vi "Obtain Broadcast Events.vi"(8 "error in":errorcluster, 10 "Create New? (F)":bool) -> (0 "error out":errorcluster, 2 "Main HMI Broadcast Events":T1)   [LabVIEW 2021, in "Main HMI.lvlib"]
doc: "This VI Obtains/Creates the Broadcast events that will be used for other modules to register to receive messages from the module that owns this VI.\n\n<b>NOTE</b>: The contents of this VI are automatically generated and modified by the <b>Tools > DQMH Consortium > DQMH</b> utilities. Consider using those utilities instead of making your own modifications to this VI.\n_____\nBased on DQMH Dev Tools: Project Template 7.1.2.1547."
uses:
  Main HMI.lvlib
  Broadcast Events--cluster.ctl
  Did Init Argument--cluster.ctl
  Status Updated Argument--cluster.ctl
  Error Reported Argument--cluster.ctl
  Stop Argument--cluster.ctl
  Get Module Execution Status Argument--cluster.ctl
panel:
  # "NOTE: The contents of this VI are automatically generated and modified by the Tools > DQMH Consortium > DQMH utilities. Consider using those utilities instead of making your own modifications to this VI."
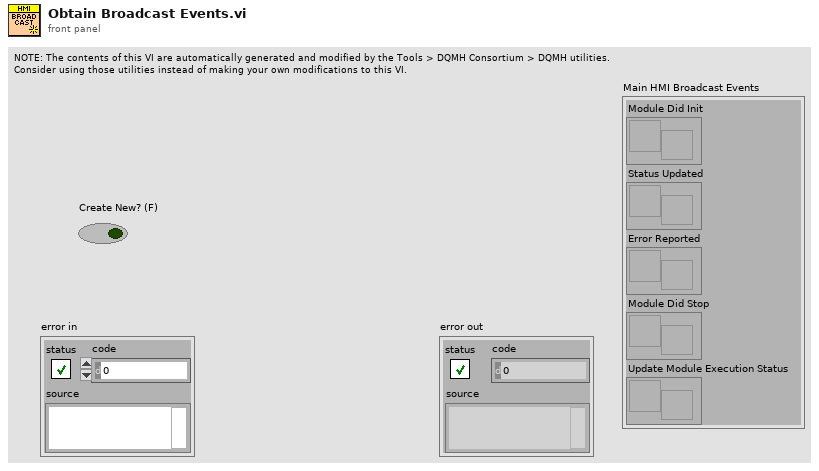
[diagram p1: front panel]
types:
  T1 = typedef "Main HMI.lvlib/Broadcast Events--cluster.ctl" = cluster{"Module Did Init":refnum<user-event>, "Status Updated":refnum<user-event>, "Error Reported":refnum<user-event>, "Module Did Stop":refnum<user-event>, "Update Module Execution Status":refnum<user-event>}
  T2 = typedef "Main HMI.lvlib/Get Module Execution Status Argument--cluster.ctl" = cluster{"Running?":bool}
  T3 = typedef "Main HMI.lvlib/Stop Argument--cluster.ctl" = cluster{"Origin":string, "Exit via Stop Module Req?":bool, "Wait for Module to stop?":bool}
  T4 = typedef "Main HMI.lvlib/Error Reported Argument--cluster.ctl" = cluster{"Error":errorcluster, "Additional Information":string, "Module Name":string}
  T5 = typedef "Main HMI.lvlib/Status Updated Argument--cluster.ctl" = cluster{"Status":string}
  T6 = typedef "Main HMI.lvlib/Did Init Argument--cluster.ctl" = cluster{"Init?":bool, "Info":string}
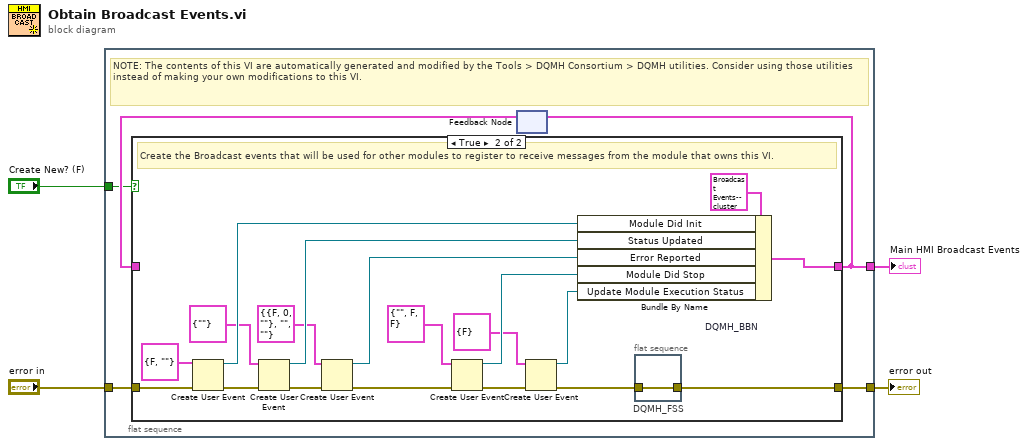
[diagram p0: block diagram]
diagram:
  n1 = flat-sequence {
    tunnel: [w9] -> w4
    tunnel: "error in" -> [w8]
    tunnel: [w6] -> w1
    tunnel: "Create New? (F)" -> [w5]
    frame #0 {
      # "NOTE: The contents of this VI are automatically generated and modified by the Tools > DQMH Consortium > DQMH utilities. Consider using those utilities instead of making your own modifications to this VI."
      n2 = feedback #1() -> (w7:T1)  [unwired: 1 in]
      n3 = case shown="True" w5 {
        tunnel: [w10 w15] -> w9
        tunnel: w8 -> [w10 w30]
        tunnel: [w11 w27] -> w6
        tunnel: w7 -> [w11 _]
        frame False {
          # "Obtain the Broadcast events that were created in a previous call to this VI."
        }
        frame True {
          # "Create the Broadcast events that will be used for other modules to register to receive messages from the module that owns this VI."
          n4 = Create User Event(user event datatype=T6 {"Init?"=FALSE, "Info"=""} ("Did Init Argument"), error in=w30) -> (user event=w28:refnum<user-event>, error out=w25:errorcluster)
          n5 = Create User Event(user event datatype=T5 {"Status"=""} ("Status Updated Argument"), error in=w25) -> (user event=w22:refnum<user-event>, error out=w24:errorcluster)
          n6 = Create User Event(user event datatype=T4 {"Error"={"status"=FALSE, "code"=0, "source"=""}, "Additional Information"="", "Module Name"=""} ("Error Reported Argument"), error in=w24) -> (user event=w19:refnum<user-event>, error out=w21:errorcluster)
          n7 = Create User Event(user event datatype=T3 {"Origin"="", "Exit via Stop Module Req?"=FALSE, "Wait for Module to stop?"=FALSE} ("Stop Argument"), error in=w21) -> (user event=w17:refnum<user-event>, error out=w16:errorcluster)
          n8 = Create User Event(user event datatype=T2 {"Running?"=FALSE} ("Get Module Execution Status Argument"), error in=w16) -> (user event=w13:refnum<user-event>, error out=w14:errorcluster)
          n9 = Bundle By Name "DQMH_BBN"(cluster=T1 {"Module Did Init"=refnum, "Status Updated"=refnum, "Error Reported"=refnum, "Module Did Stop"=refnum, "Update Module Execution Status"=refnum} ("output cluster"), "Module Did Init"=w28, "Status Updated"=w22, "Error Reported"=w19, "Module Did Stop"=w17, "Update Module Execution Status"=w13) -> (w27:T1)
          n10 = flat-sequence "DQMH_FSS" {
            tunnel: w14 -> [w31]
            tunnel: [w31] -> w15
            frame #0 {
            }
          }
        }
      }
      n11 = feedback-in #1(w6) -> ()
    }
  }
  "error out" <- w4
  "Main HMI Broadcast Events" <- w1
